vi "Test_settings_fifo.vi"() -> ()   [LabVIEW 2013]
uses:
  <vilib>/userdefined/High Color/nirio_resource_hc.ctl
  Config/FPGAref_config.ctl
  FPGA/fpga_settings.ctl
  <vilib>/FPGAPlugInAG/PXIe-7975R/niLvFpga_Open_PXIe-7975R.vi
  <vilib>/rvi/interface/common/dynamic/niFpgaDynamicAddResources.vi
  <vilib>/rvi/interface/common/niFpgaWaitOnOcc.vi
  <vilib>/Utility/error.llb/Error Cluster From Error Code.vi
  <vilib>/rvi/errors/niLvFpgaAdjustHostInterfaceError.vi
  <vilib>/rvi/interface/nirviOpenFPGA/nirviOpenFPGA.xnode
  FPGA Bitfiles/delaytest2_0waIOfTFc3I.lvbitx
  <vilib>/rvi/interface/nirviMethod/nirviMethod.xnode
  <vilib>/rvi/FXPMathLib/FxpInterpret/XNode/nifxpmath_Interpret.xnode
  <vilib>/rvi/interface/nirviReadWriteControl/nirviReadWriteControl.xnode
  <vilib>/FPGAPlugInAG/Dynamic/niLvFpga_WriteFifo_Dynamic.vi
  <vilib>/rvi/errors/niLvFpgaMergeErrorWithErrorCode.vi
  NiFpgaLv.dll
  <vilib>/rvi/interface/Simulation/niFpgaSimulationCallBeginRW.vi
  <vilib>/FPGAPlugInAG/Dynamic/niLvFpga_ConfigureFifo_Dynamic.vi
  <vilib>/FPGAPlugInAG/Dynamic/niLvFpga_StartFifo_Dynamic.vi
panel:
  in  "Output delay delta 2":dbl(slide) scale=0.0..6.0
  out "fixed-point 3":fxp<+/-,32,4>
  in  "Output delay 2":dbl(slide) scale=0.0..6.0
  out "fixed-point 4":fxp<+/-,32,4>
  out "Actual Depth":u32
  in  "stop":bool
  out "fixed-point 2":fxp<+/-,32,4>
  out "fixed-point":fxp<+/-,32,4>
  out "Fi_delta":fxp<+/-,32,4>
  out "Fi_start":fxp<+/-,32,4>
  out "error out 2":errorcluster
  in  "Output delay delta":dbl(slide) scale=0.0..6.0
  in  "Output delay":dbl(slide) scale=0.0..6.0
  in  "Mixer freq [MHz]":dbl
  out "Configured?":bool
  out "Clocking Option Configured?":bool
  in  "resource name":T1="PXI1Slot18"
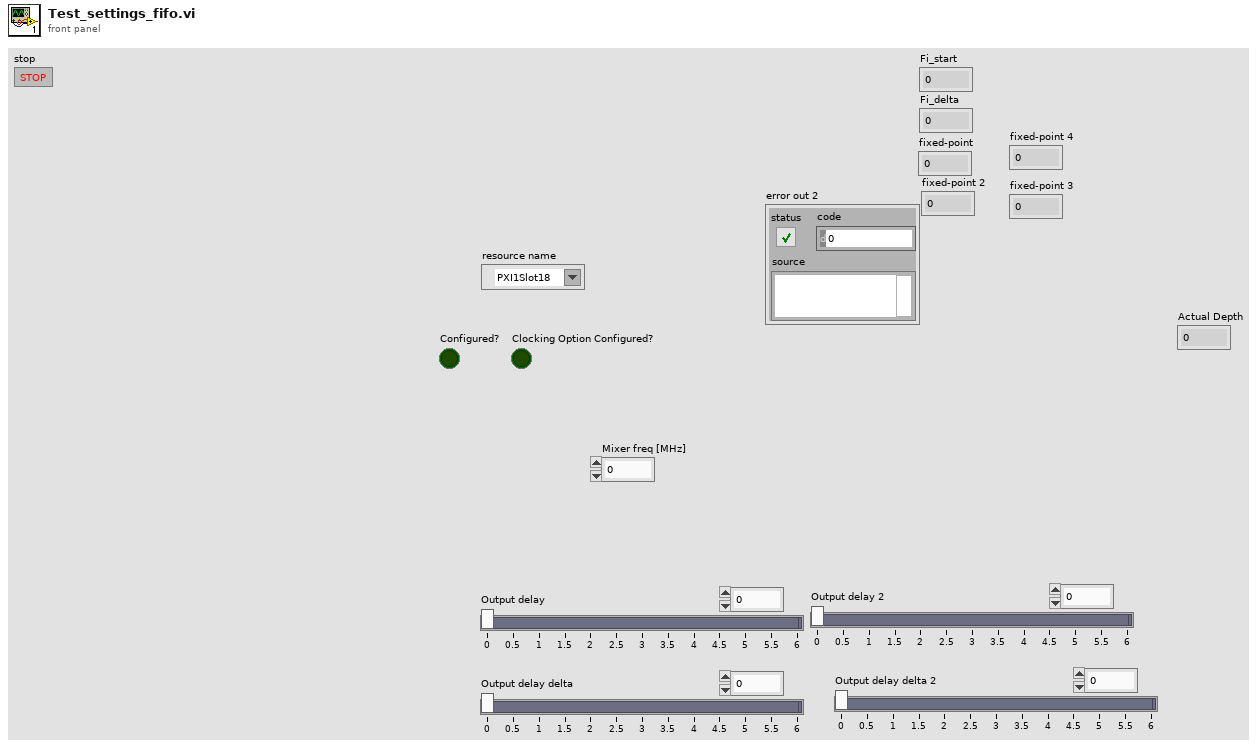
[diagram p1: front panel]
types:
  T1 = typedef "nirio_resource_hc.ctl" = tag
  T2 = typedef "FPGAref_config.ctl" = refnum<k20>
  T3 = enum8{"Internal Clock PLL Off", "Internal Clock PLL On (REF IN)", "External Clock (CLK_IN)", "Internal Clock PLL On (IoModSyncClk)"}
  T4 = typedef "FPGAref_5782.ctl" = refnum<k20>
  T5 = typedef "fpga_settings.ctl" = enum16{"Feedback Enable", "New FIR coeffs", "FIR shift", "Enable filter", "Set Downsample", "Downsample", "CIC Gain", "Record length", "Trigger samples", "Quiet time", "a_am", "b_am", "Use fixed delay", "fixed sin_fi", "fixed cos_fi", "Ki*Tau", "Kp", "Kd_Tau", "Fi_start", "Fi_delta", "DC_offs 0", "DC_offs 1", "DC_offs 2", "DC_offs 3", "Ki*Tau am", "Kp am", "Kd_Tau am", "Feedback AM"}
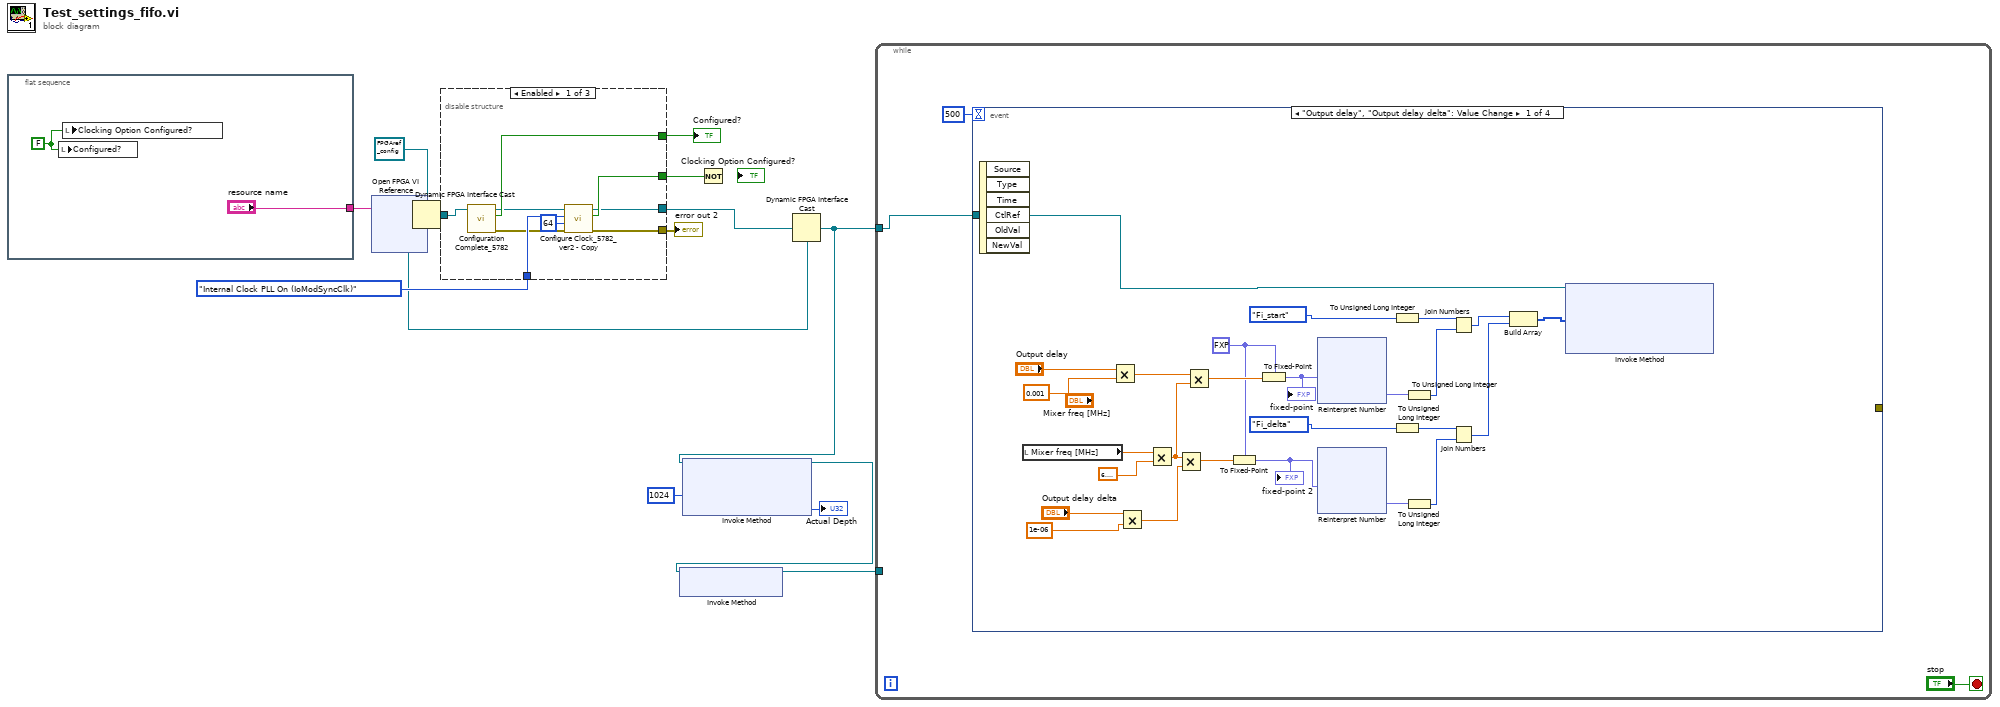
[diagram p0: block diagram]
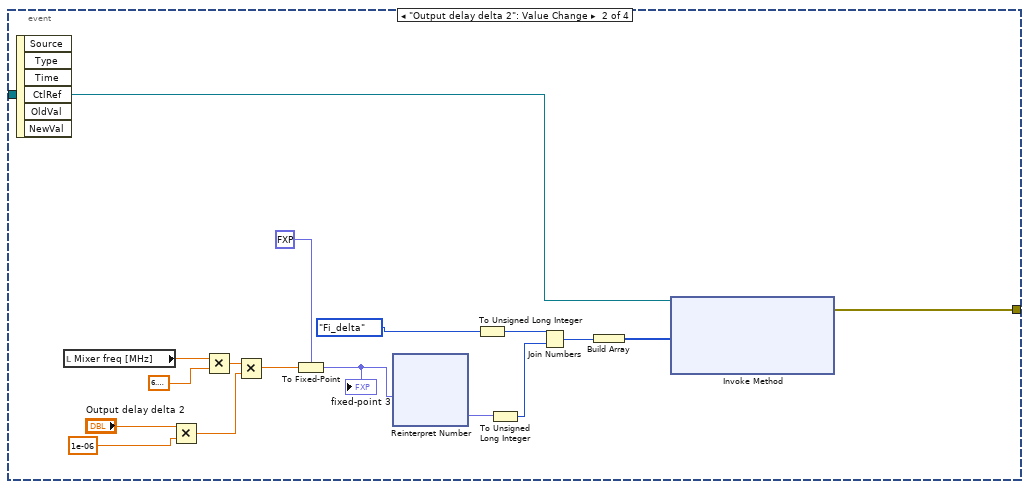
[diagram p2: hidden frame]
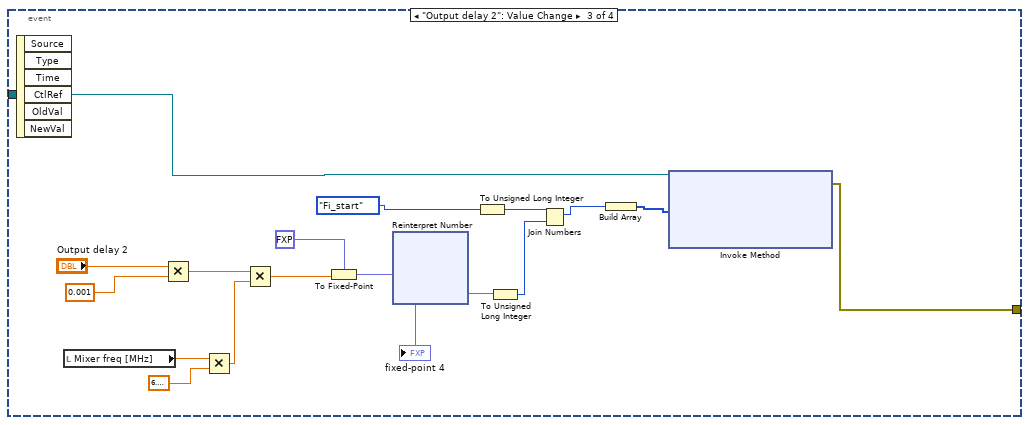
[diagram p3: hidden frame]
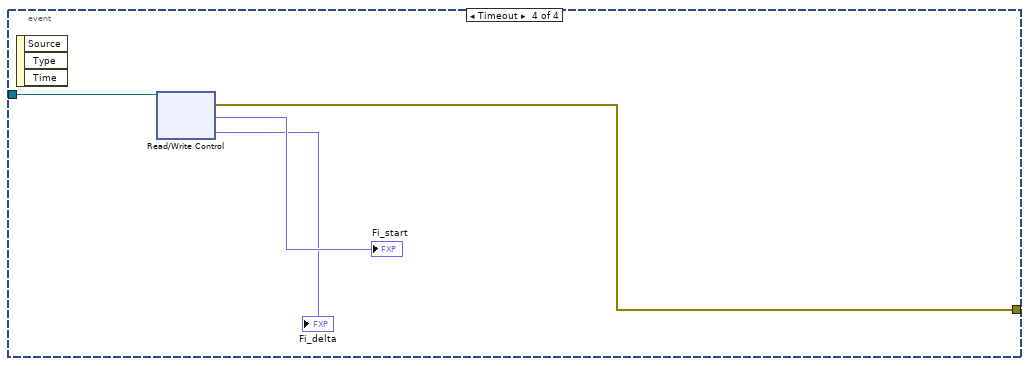
[diagram p4: hidden frame]
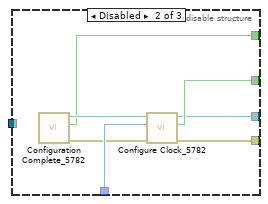
[diagram p5: hidden frame]
diagram:
  n1 = flat-sequence {
    tunnel: ["resource name"] -> w14
    frame #0 {
      w15 = FALSE ("Trigger Acquisition")
      n2 = local write "Configured?"(w15) -> ()
      n3 = local write "Clocking Option Configured?"(w15) -> ()
    }
  }
  n4 = xnode "Open FPGA VI Reference"("resource name"=w14) -> ("FPGA VI Reference Out"=w8:refnum<k20>)  [unwired: 1 in, 1 out]
  n5 = Dynamic FPGA Interface Cast(Session In=T2 refnum ("FPGA VI Reference in"), Type=w8) -> (Session Out=w10:T2)
  n6 = disable-structure shown="Enabled" {
    disable-tunnel: [w25 w32 _] -> w13
    disable-tunnel: T3."Internal Clock PLL On (IoModSyncClk)" ("Clock Source") -> [w24 w31 _]
    disable-tunnel: [w22 w29 _] -> w6
    disable-tunnel: [w21 w27 w33] -> w7
    disable-tunnel: [w20 w26 _] -> w12
    disable-tunnel: w10 -> [w17 _ _]
    frame Enabled {
      n7 = call "Configuration Complete_5782.vi"("FPGA VI Reference in"=w17) -> ("error out"=w23:errorcluster, "Configured?"=w20:bool, "FPGA VI Reference out"=w19:T2)  [unwired: 8 in]
      n8 = call "Configure Clock_5782_ver2 - Copy.vi"("error in"=w23, "User Data 1"=u8 64, "Clock Source"=w24, "FPGA VI Reference"=w19) -> ("error out"=w22:errorcluster, "Configuration Error"=w25:bool, "FPGA VI Reference out"=w21:T2)  [unwired: 5 in]
    }
    frame Disabled {
      n9 = call "Configuration Complete_5782.vi"() -> ("error out"=w30:errorcluster, "Configured?"=w26:bool, "FPGA VI Reference out"=w28:T2)  [unwired: 9 in]
      n10 = call "Configure Clock_5782.vi"("error in"=w30, "Clock Source"=w31, "FPGA VI Reference in"=w28) -> ("error out"=w29:errorcluster, "Configuration Error"=w32:bool, "FPGA VI Reference Out"=w27:T4)  [unwired: 6 in]
    }
    frame Disabled {
    }
  }
  "Configured?" <- w12
  "error out 2" <- w6
  n11 = Not(x=w13) -> ()  [unwired: 1 out]
  n12 = Dynamic FPGA Interface Cast(Session In=w8, Type=w7) -> (Session Out=w5:refnum<k20>)
  n13 = xnode "Invoke Method"("FPGA VI Reference In"=w5, "Requested Depth"=u32 1024) -> ("FPGA VI Reference Out"=w2:refnum<k20>, "Actual Depth"=→"Actual Depth":u32)  [unwired: 1 in, 1 out]
  n14 = xnode "Invoke Method"("FPGA VI Reference In"=w2) -> ("FPGA VI Reference Out"=w1:refnum<k20>)  [unwired: 1 in, 1 out]
  n15 = while {
    tunnel: w5 -> [w36]
    tunnel: w1 -> [_]
    stop <- "stop" stop-if-true
    n16 = event shown="[0] \"Output delay\", \"Output delay delta\": Value Change" {
      selector: _ -> [_ _ _ _]
      dyn-events: _ -> [_ _ _ _]
      timeout: 500 -> [_ _ _ _]
      tunnel: w36 -> [w40 w65 w83 w100]
      tunnel: [_ w63 w80 w97] -> _
      event "Output delay", "Output delay delta": Value Change {
        w42 = fxp<+/-,32,4> 0.0 ("x")
        n17 = event-data() -> ()  [unwired: 1 in, 6 out]
        n18 = local read "Mixer freq [MHz]"() -> (w56:dbl)
        n19 = Multiply(x="Output delay", y=0.001) -> (x*y=w57:dbl)
        n20 = Multiply(x="Output delay delta", y=1e-06) -> (x*y=w59:dbl)
        n21 = Multiply(x=w56, y=6.283185307179586) -> (x*y=w54:dbl)
        n22 = Multiply(x=w54, y=w59) -> (x*y=w43:dbl)
        n23 = Multiply(x=w57, y=w54) -> (x*y=w45:dbl)
        n24 = To Fixed-Point(fixed-point type=w42, number=w43) -> (fixed-point=w41:fxp<+/-,32,4>)
        "fixed-point 2" <- w41
        n25 = To Fixed-Point(fixed-point type=w42, number=w45) -> (fixed-point=w44:fxp<+/-,32,4>)
        "fixed-point" <- w44
        n26 = xnode "Reinterpret Number"("x"=w44) -> ("y"=w50:fxp<+,32,32>)
        n27 = xnode "Reinterpret Number"("x"=w41) -> ("y"=w49:fxp<+,32,32>)
        n28 = To Unsigned Long Integer(number=fpga_settings."Fi_start" ("FPGA Setting")) -> (unsigned 32bit integer=w53:u32)
        n29 = To Unsigned Long Integer(number=fpga_settings."Fi_delta" ("FPGA Setting")) -> (unsigned 32bit integer=w46:u32)
        n30 = To Unsigned Long Integer(number=w50) -> (unsigned 32bit integer=w52:u32)
        n31 = To Unsigned Long Integer(number=w49) -> (unsigned 32bit integer=w47:u32)
        n32 = Join Numbers(hi=w53, lo=w52) -> ((hi.lo)=w39:u64)
        n33 = Join Numbers(hi=w46, lo=w47) -> ((hi.lo)=w37:u64)
        n34 = Build Array(w39, w37) -> (w38:u64[])
        n35 = xnode "Invoke Method"("FPGA VI Reference In"=w40, "Data"=w38) -> ()  [unwired: 2 in, 3 out]
      }
      event "Output delay delta 2": Value Change {
        n36 = event-data() -> ()  [unwired: 1 in, 6 out]
        n37 = local read "Mixer freq [MHz]"() -> (w76:dbl)
        n38 = Multiply(x="Output delay delta 2", y=1e-06) -> (x*y=w78:dbl)
        n39 = Multiply(x=w76, y=6.283185307179586) -> (x*y=w74:dbl)
        n40 = Multiply(x=w74, y=w78) -> (x*y=w69:dbl)
        n41 = To Fixed-Point(fixed-point type=fxp<+/-,32,4> 0.0 ("x"), number=w69) -> (fixed-point=w67:fxp<+/-,32,4>)
        "fixed-point 3" <- w67
        n42 = xnode "Reinterpret Number"("x"=w67) -> ("y"=w73:fxp<+,32,32>)
        n43 = To Unsigned Long Integer(number=fpga_settings."Fi_delta" ("FPGA Setting")) -> (unsigned 32bit integer=w70:u32)
        n44 = To Unsigned Long Integer(number=w73) -> (unsigned 32bit integer=w71:u32)
        n45 = Join Numbers(hi=w70, lo=w71) -> ((hi.lo)=w64:u64)
        n46 = Build Array(w64) -> (w66:u64[])
        n47 = xnode "Invoke Method"("FPGA VI Reference In"=w65, "Data"=w66) -> ("error out"=w63:errorcluster)  [unwired: 2 in, 2 out]
      }
      event "Output delay 2": Value Change {
        n48 = event-data() -> ()  [unwired: 1 in, 6 out]
        n49 = local read "Mixer freq [MHz]"() -> (w92:dbl)
        n50 = Multiply(x="Output delay 2", y=0.001) -> (x*y=w93:dbl)
        n51 = Multiply(x=w92, y=6.283185307179586) -> (x*y=w91:dbl)
        n52 = Multiply(x=w93, y=w91) -> (x*y=w86:dbl)
        n53 = To Fixed-Point(fixed-point type=fxp<+/-,32,4> 0.0 ("x"), number=w86) -> (fixed-point=w85:fxp<+/-,32,4>)
        "fixed-point 4" <- w85
        n54 = xnode "Reinterpret Number"("x"=w85) -> ("y"=w87:fxp<+,32,32>)
        n55 = To Unsigned Long Integer(number=fpga_settings."Fi_start" ("FPGA Setting")) -> (unsigned 32bit integer=w90:u32)
        n56 = To Unsigned Long Integer(number=w87) -> (unsigned 32bit integer=w89:u32)
        n57 = Join Numbers(hi=w90, lo=w89) -> ((hi.lo)=w81:u64)
        n58 = Build Array(w81) -> (w82:u64[])
        n59 = xnode "Invoke Method"("FPGA VI Reference In"=w83, "Data"=w82) -> ("error out"=w80:errorcluster)  [unwired: 2 in, 2 out]
      }
      event Timeout {
        n60 = event-data() -> ()  [unwired: 1 in, 3 out]
        n61 = xnode "Read/Write Control"("FPGA VI Reference In"=w100) -> ("error out"=w97:errorcluster, "Fi_start"=→"Fi_start":fxp<+/-,32,4>, "Fi_delta"=→"Fi_delta":fxp<+/-,32,4>)  [unwired: 1 in, 1 out]
      }
    }
  }
